vi "SeqMap_Read.vi"(8 "error in (no error)":errorcluster, 11 "Tag":string) -> (0 "Error Out":errorcluster, 2 "Found?":bool, 3 "Value":variant)   [LabVIEW 2016, in "SeqProcessor.lvlib"]
uses:
  SeqProcessor.lvlib
  <vilib>/addons/PointValueMap/subVIs/Point_Read_variant.vi
  <vilib>/addons/PointValueMap/PointValueMap.lvlib
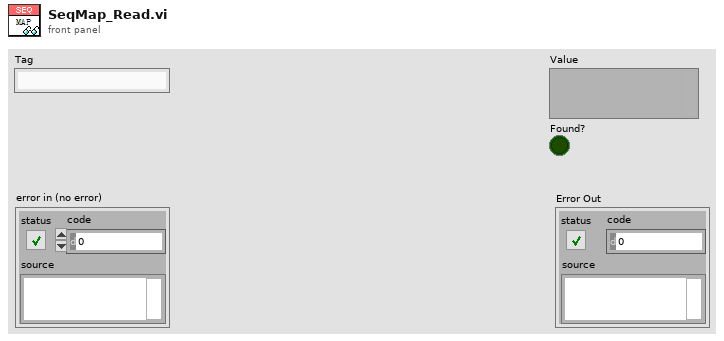
[diagram p1: front panel]
types:
  T1 = typedef "PointValueMap.lvlib/PointMap.ctl" = refnum<data-value>
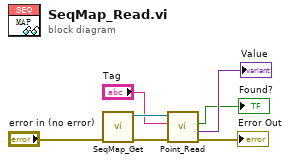
[diagram p0: block diagram]
diagram:
  n1 = call "SeqMap_Get.vi"("error in (no error)"="error in (no error)") -> ("error out"=w7:errorcluster, "SeqMap"=w6:T1)  [unwired: 9 in]
  n2 = call-poly <vilib>:"Point_Read.vi"("Error In"=w7, "Tag"="Tag", "Map"=w6) -> ("Error Out"=→"Error Out":errorcluster, "Value"=→"Value":variant, "Found?"=→"Found?":bool)  [unwired: 3 in, 3 out]
